vi "LC Show Control.vi"(8 "error in (no error)":errorcluster caption="Error In") -> (0 "error out":errorcluster caption="Error Out")   [LabVIEW 2020]
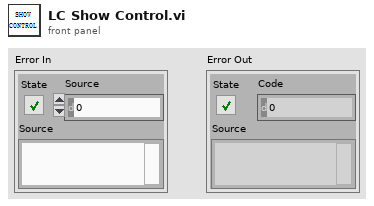
[diagram p1: front panel]
types:
  T1 = typedef "LVBoundsTypeDef.ctl" = cluster{"Width":u32, "Height":u32}
  T2 = typedef "LVPositionTypeDef.ctl" = cluster{"Left":i32, "Top":i32}
  T3 = typedef "LVRowAndColumnTypeDef.ctl" = cluster{"Row":i32, "Column":i32}
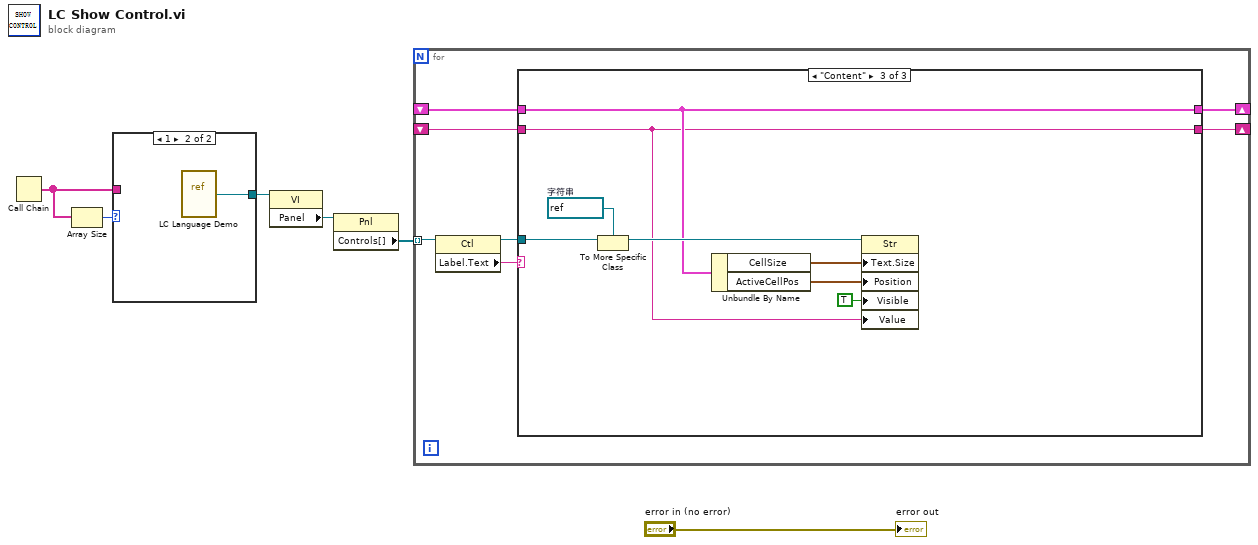
[diagram p0: block diagram]
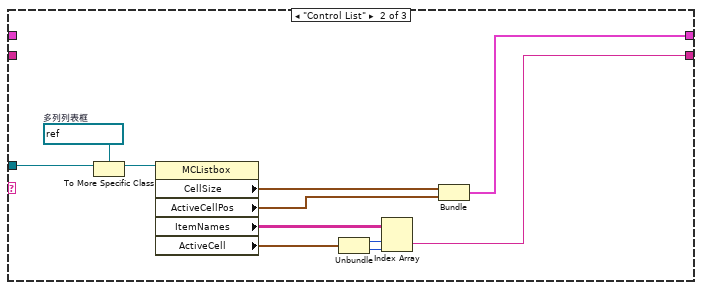
[diagram p3: hidden frame]
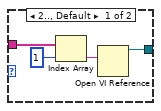
[diagram p4: hidden frame]
diagram:
  n1 = Call Chain() -> (call chain=w3:string[])
  n2 = Array Size(array=w3) -> (size(s)=w4:i32)
  n3 = case shown="1" w4 {
    tunnel: [w8 w11] -> w1
    tunnel: w3 -> [w7 _]
    frame 2.., Default {
      n4 = Index Array(array=w7, index=1 ("索引")) -> (element=w9:string)
      n5 = Open VI Reference(vi path=w9) -> (vi reference=w8:refnum<vi>)  [unwired: 5 in, 1 out]
    }
    frame 1 {
      n6 = vi-ref "LC Language Demo.vi"() -> (w11:refnum<vi>)
    }
  }
  n7 = property class="VI"(reference=w1) -> ("Panel"=w2:refnum<vi>)  [unwired: 1 in, 2 out]
  n8 = property class="Pnl"(reference=w2) -> ("Controls[]"=w5:refnum<vi>[])  [unwired: 1 in, 2 out]
  n9 = for {
    tunnel: w5 -> [w18] mode=indexing
    shift-right: [w15] -> _
    shift-left: _ -> [w14]
    shift-right: [w13] -> _
    shift-left: _ -> [w12]
    n10 = property class="Ctl"(reference=w18) -> (reference out=w16:refnum<vi>, "Label.Text"=w17:string)  [unwired: 1 in, 1 out]
    n11 = case shown="\"Content\"" w17 {
      tunnel: w16 -> [_ w31 w39]
      tunnel: [w20 w26 w36] -> w15
      tunnel: w14 -> [w20 _ w36]
      tunnel: [w19 w21 w32] -> w13
      tunnel: w12 -> [w19 _ w32]
      frame "eee", Default {
      }
      frame "Control List" {
        w29 = refnum<vi> refnum  # 多列列表框
        n12 = To More Specific Class(target class=w29, reference=w31) -> (specific class reference=w30:refnum<vi>)  [unwired: 1 in, 1 out]
        n13 = property class="MCListbox"(reference=w30) -> ("CellSize"=w28:T1, "ActiveCellPos"=w27:T2, "ItemNames"=w25:string[][], "ActiveCell"=w24:T3)  [unwired: 1 in, 2 out]
        n14 = Unbundle(w24) -> ("Row"=w23:i32, "Column"=w22:i32)
        n15 = Index Array(array=w25, index (row)=w23, index (col)=w22) -> (element=w21:string)
        n16 = Bundle("CellSize"=w28, "ActiveCellPos"=w27) -> (w26:cluster{"CellSize":T1, "ActiveCellPos":T2})  [unwired: 1 in]
      }
      frame "Content" {
        w38 = refnum<vi> refnum  # 字符串
        n17 = To More Specific Class(target class=w38, reference=w39) -> (specific class reference=w37:refnum<vi>)  [unwired: 1 in, 1 out]
        n18 = Unbundle By Name(w36) -> ("CellSize"=w34:T1, "ActiveCellPos"=w35:T2)
        n19 = property class="Str"(reference=w37, "Text.Size"=w34, "Position"=w35, "Visible"=TRUE ("可见"), "Value"=w32) -> ()  [unwired: 1 in, 2 out]
      }
    }
  }
  "error out" <- "error in (no error)"
